vi "pt2xy.vi"(6 "history for statistics (100)":i32=100 format="%.0p", 7 "reset?":bool, 8 "history to keep (10k)":i32=10000 format="%.0p", 9 "history to display (1k)":i32=1000 format="%.0p", 10 "dt from last data point":dbl format="%.2p s", 11 "input data point":variant) -> (1 "history for statistics":cluster{dbl[], dbl[]}, 2 "dt out":dbl format="%#_6p s", 3 "waveform":cluster{dbl[], dbl[]}(graph) caption="xy graph")   [LabVIEW 2015]
uses:
  poly_data_queue_double.vi
  <vilib>/ptbypt/NI_PtbyPt.lvlib
  <vilib>/Utility/Data Type/NI_Data Type.lvlib
  _average_tools_polys.lvlib
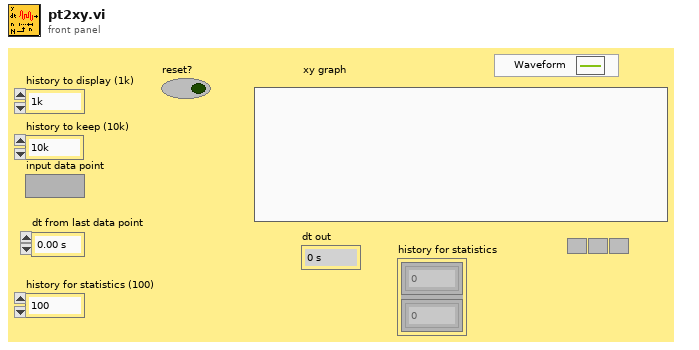
[diagram p1: front panel]
types:
  T1 = typedef "LVNumericRepresentation.ctl" = enum32{"Extended Precision", "Double Precision", "Single Precision", "Long", "Word", "Byte", "Unsigned Long", "Unsigned Word", "Unsigned Byte", "Complex Extended", "Complex Double", "Complex Single", "Quad", "Unsigned Quad", "Fixed-Point"}
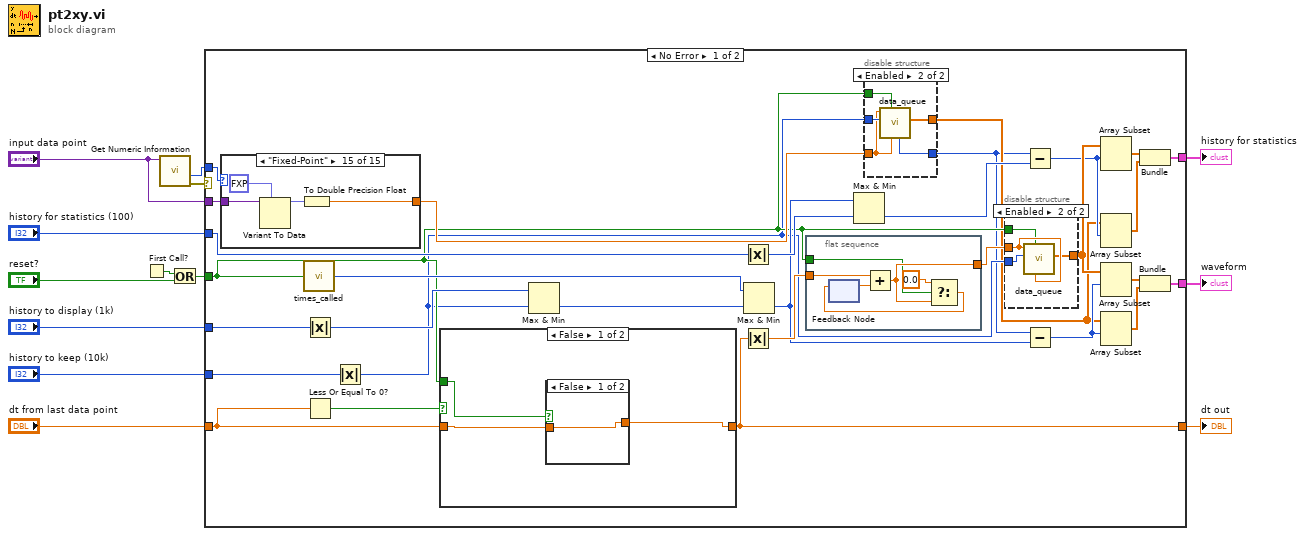
[diagram p0: block diagram]
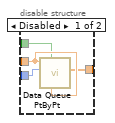
[diagram p2: hidden frame]
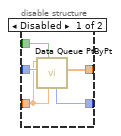
[diagram p3: hidden frame]
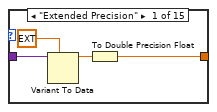
[diagram p4: hidden frame]
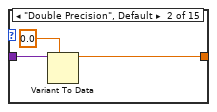
[diagram p5: hidden frame]
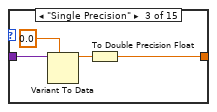
[diagram p6: hidden frame]
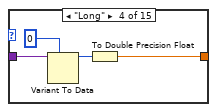
[diagram p7: hidden frame]
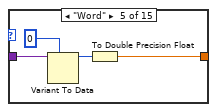
[diagram p8: hidden frame]
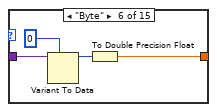
[diagram p9: hidden frame]
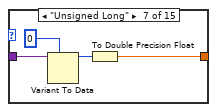
[diagram p10: hidden frame]
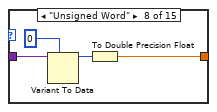
[diagram p11: hidden frame]
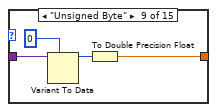
[diagram p12: hidden frame]
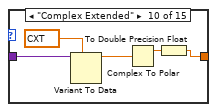
[diagram p13: hidden frame]
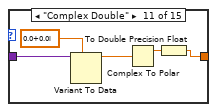
[diagram p14: hidden frame]
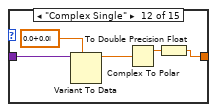
[diagram p15: hidden frame]
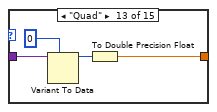
[diagram p16: hidden frame]
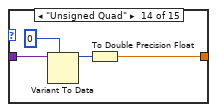
[diagram p17: hidden frame]
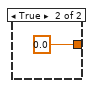
[diagram p18: hidden frame]
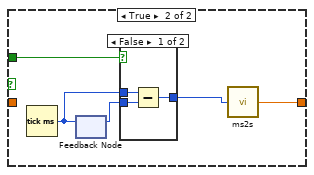
[diagram p19: hidden frame]
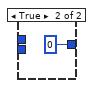
[diagram p20: hidden frame]
diagram:
  n1 = First Call?() -> (First Call?: T/F=w3:bool)
  n2 = call <vilib>:"Get Numeric Information.vi"("Variant"="input data point") -> ("error out"=w9:errorcluster, "Representation"=w7:T1)  [unwired: 7 in, 2 out]
  n3 = Or(x=w3, y="reset?") -> (x .or. y?=w4:bool)
  n4 = case shown="No Error" w9 {
    tunnel: "history to display (1k)" -> [w42 _]
    tunnel: "history to keep (10k)" -> [w40 _]
    tunnel: "dt from last data point" -> [w36 w144]
    tunnel: w4 -> [w17 _]
    tunnel: [w35 w144] -> w10
    tunnel: "input data point" -> [w33 _]
    tunnel: w7 -> [w34 _]
    tunnel: [w31 _] -> w6
    tunnel: "history for statistics (100)" -> [w30 _]
    tunnel: [w21 _] -> w1
    frame No Error {
      n5 = case shown="\"Fixed-Point\"" w34 {
        tunnel: w33 -> [w64 w68 w72 w76 w78 w82 w86 w90 w94 w100 w103 w108 w113 w117 w121]
        tunnel: [w62 w66 w69 w73 w77 w81 w85 w89 w93 w97 w102 w107 w112 w116 w120] -> w18
        frame "Extended Precision" {
          n6 = Variant To Data(type=ext 0.0, Variant=w64) -> (data=w63:ext)  [unwired: 1 in, 1 out]
          n7 = To Double Precision Float(number=w63) -> (double precision float=w62:dbl)
        }
        frame "Double Precision", Default {
          n8 = Variant To Data(type=0.0, Variant=w68) -> (data=w66:dbl)  [unwired: 1 in, 1 out]
        }
        frame "Single Precision" {
          n9 = Variant To Data(type=sgl 0.0, Variant=w72) -> (data=w70:sgl)  [unwired: 1 in, 1 out]
          n10 = To Double Precision Float(number=w70) -> (double precision float=w69:dbl)
        }
        frame "Long" {
          n11 = Variant To Data(type=0, Variant=w76) -> (data=w74:i32)  [unwired: 1 in, 1 out]
          n12 = To Double Precision Float(number=w74) -> (double precision float=w73:dbl)
        }
        frame "Word" {
          n13 = Variant To Data(type=i16 0, Variant=w78) -> (data=w79:i16)  [unwired: 1 in, 1 out]
          n14 = To Double Precision Float(number=w79) -> (double precision float=w77:dbl)
        }
        frame "Byte" {
          n15 = Variant To Data(type=i8 0, Variant=w82) -> (data=w83:i8)  [unwired: 1 in, 1 out]
          n16 = To Double Precision Float(number=w83) -> (double precision float=w81:dbl)
        }
        frame "Unsigned Long" {
          n17 = Variant To Data(type=u32 0, Variant=w86) -> (data=w87:u32)  [unwired: 1 in, 1 out]
          n18 = To Double Precision Float(number=w87) -> (double precision float=w85:dbl)
        }
        frame "Unsigned Word" {
          n19 = Variant To Data(type=u16 0, Variant=w90) -> (data=w91:u16)  [unwired: 1 in, 1 out]
          n20 = To Double Precision Float(number=w91) -> (double precision float=w89:dbl)
        }
        frame "Unsigned Byte" {
          n21 = Variant To Data(type=u8 0, Variant=w94) -> (data=w95:u8)  [unwired: 1 in, 1 out]
          n22 = To Double Precision Float(number=w95) -> (double precision float=w93:dbl)
        }
        frame "Complex Extended" {
          n23 = Variant To Data(type=cxt 0.0+0.0i, Variant=w100) -> (data=w99:cxt)  [unwired: 1 in, 1 out]
          n24 = Complex To Polar(r * e^(i*theta)=w99) -> (r=w98:ext)  [unwired: 1 out]
          n25 = To Double Precision Float(number=w98) -> (double precision float=w97:dbl)
        }
        frame "Complex Double" {
          n26 = Variant To Data(type=cdb 0.0+0.0i, Variant=w103) -> (data=w105:cdb)  [unwired: 1 in, 1 out]
          n27 = Complex To Polar(r * e^(i*theta)=w105) -> (r=w104:dbl)  [unwired: 1 out]
          n28 = To Double Precision Float(number=w104) -> (double precision float=w102:dbl)
        }
        frame "Complex Single" {
          n29 = Variant To Data(type=csg 0.0+0.0i, Variant=w108) -> (data=w110:csg)  [unwired: 1 in, 1 out]
          n30 = Complex To Polar(r * e^(i*theta)=w110) -> (r=w109:sgl)  [unwired: 1 out]
          n31 = To Double Precision Float(number=w109) -> (double precision float=w107:dbl)
        }
        frame "Quad" {
          n32 = Variant To Data(type=i64 0, Variant=w113) -> (data=w114:i64)  [unwired: 1 in, 1 out]
          n33 = To Double Precision Float(number=w114) -> (double precision float=w112:dbl)
        }
        frame "Unsigned Quad" {
          n34 = Variant To Data(type=u64 0, Variant=w117) -> (data=w118:u64)  [unwired: 1 in, 1 out]
          n35 = To Double Precision Float(number=w118) -> (double precision float=w116:dbl)
        }
        frame "Fixed-Point" {
          n36 = Variant To Data(type=fxp<+,1,1> 0.0, Variant=w121) -> (data=w122:fxp<+,1,1>)  [unwired: 1 in, 1 out]
          n37 = To Double Precision Float(number=w122) -> (double precision float=w120:dbl)
        }
      }
      n38 = call "times_called.vi"("reset?"=w17) -> ("times called"=w43:i32)  [unwired: 8 in]
      n39 = Absolute Value(x=w42) -> (abs(x)=w41:i32)
      n40 = Less Or Equal To 0?(x=w36) -> (x <= 0?=w37:bool)
      n41 = Absolute Value(x=w40) -> (abs(x)=w16:i32)
      n42 = case shown="False" w37 {
        tunnel: [w125 w130] -> w35
        tunnel: w36 -> [w124 _]
        tunnel: w17 -> [w126 w133]
        frame False {
          n43 = case shown="False" w126 {
            tunnel: [w127 0.0 ("t")] -> w125
            tunnel: w124 -> [w127 _]
            frame False {
            }
            frame True {
            }
          }
        }
        frame True {
          n44 = Tick Count (ms)() -> (millisecond timer value=w129:u32)
          n45 = feedback #1() -> (w132:u32)  [unwired: 1 in]
          n46 = feedback-in #1(w129) -> ()
          n47 = case shown="False" w133 {
            tunnel: [w136 u32 0] -> w131
            tunnel: w132 -> [w135 _]
            tunnel: w129 -> [w134 _]
            frame False {
              n48 = Subtract(x=w134, y=w135) -> (x-y=w136:u32)
            }
            frame True {
            }
          }
          n49 = call "ms2s.vi"("ms"=w131) -> ("s"=w130:dbl)  [unwired: 4 in]
        }
      }
      n50 = Max & Min(x=w41, y=w16) -> (min(x,y)=w26:i32)  [unwired: 1 out]
      n51 = Absolute Value(x=w30) -> (abs(x)=w28:i32)
      n52 = Absolute Value(x=w35) -> (abs(x)=w38:dbl)
      n53 = Max & Min(x=w43, y=w26) -> (min(x,y)=w19:i32)  [unwired: 1 out]
      n54 = flat-sequence {
        tunnel: [w141] -> w39
        tunnel: w17 -> [w140]
        tunnel: w38 -> [w138]
        frame #0 {
          n55 = feedback #2() -> (w143:dbl)  [unwired: 1 in]
          n56 = Add(x=w138, y=w143) -> (x+y=w141:dbl)
          n57 = Select(t=0.0, s=w140, f=w141) -> (s? t:f=w139:dbl)
          n58 = feedback-in #2(w139) -> ()
        }
      }
      n59 = Max & Min(x=w19, y=w28) -> (min(x,y)=w20:i32)  [unwired: 1 out]
      n60 = disable-structure shown="Enabled" {
        disable-tunnel: w18 -> [w52 w59]
        disable-tunnel: w17 -> [w56 w61]
        disable-tunnel: w16 -> [w55 w60]
        disable-tunnel: [w54 w58] -> w15
        disable-tunnel: [w53 w57] -> w14
        frame Disabled {
          n61 = call <vilib>:"Data Queue PtByPt.vi"("initial queue element"=w52, "initialize"=w56, "sample length"=w55, "input data point"=w52) -> ("Current Queue"=w54:dbl[], "current length"=w53:i32)  [unwired: 3 in, 3 out]
        }
        frame Enabled {
          n62 = call-poly "data_queue.vi"("initial queue element (NaN)"=w59, "initialize"=w61, "sample length"=w60, "input data point"=w59) -> ("Queue"=w58:dbl[], "current length"=w57:i32)  [unwired: 4 in, 2 out]
        }
      }
      n63 = disable-structure shown="Enabled" {
        disable-tunnel: w39 -> [w47 w51]
        disable-tunnel: [w46 w48] -> w25
        disable-tunnel: w17 -> [w45 w49]
        disable-tunnel: w16 -> [w44 w50]
        frame Disabled {
          n64 = call <vilib>:"Data Queue PtByPt.vi"("initial queue element"=w47, "initialize"=w45, "sample length"=w44, "input data point"=w47) -> ("Current Queue"=w46:dbl[])  [unwired: 3 in, 4 out]
        }
        frame Enabled {
          n65 = call-poly "data_queue.vi"("initial queue element (NaN)"=w51, "initialize"=w49, "sample length"=w50, "input data point"=w51) -> ("Queue"=w48:dbl[])  [unwired: 4 in, 3 out]
        }
      }
      n66 = Subtract(x=w14, y=w20) -> (x-y=w24:i32)
      n67 = Subtract(x=w14, y=w19) -> (x-y=w29:i32)
      n68 = Array Subset(array=w25, index=w24) -> (w23:dbl[])  [unwired: 1 in]
      n69 = Array Subset(array=w15, index=w24) -> (w22:dbl[])  [unwired: 1 in]
      n70 = Array Subset(array=w25, index=w29) -> (w32:dbl[])  [unwired: 1 in]
      n71 = Array Subset(array=w15, index=w29) -> (w27:dbl[])  [unwired: 1 in]
      n72 = Bundle(w23, w22) -> (w21:cluster{dbl[], dbl[]})  [unwired: 1 in]
      n73 = Bundle(w32, w27) -> (w31:cluster{dbl[], dbl[]})  [unwired: 1 in]
    }
    frame Error {
      (unwired) nan ("mean")
    }
  }
  "waveform" <- w6
  "dt out" <- w10
  "history for statistics" <- w1
